vi "Read Command Error.vi"(8 "error in (no error)":errorcluster, 11 "VISA resource name":refnum<visa-resource-name>) -> (0 "error out":errorcluster, 1 "Error Message":string, 2 "Error Code":i32, 3 "VISA resource name out":refnum<visa-resource-name>)   [LabVIEW 2013, in "LeCroy Wave Series.lvlib"]
doc: "Reads and clears the contents of the Command error Register which specifies the last syntax error type detected by your oscilloscope."
uses:
  LeCroy Wave Series.lvlib
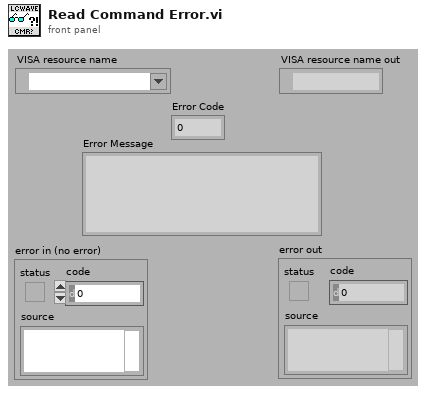
[diagram p1: front panel]
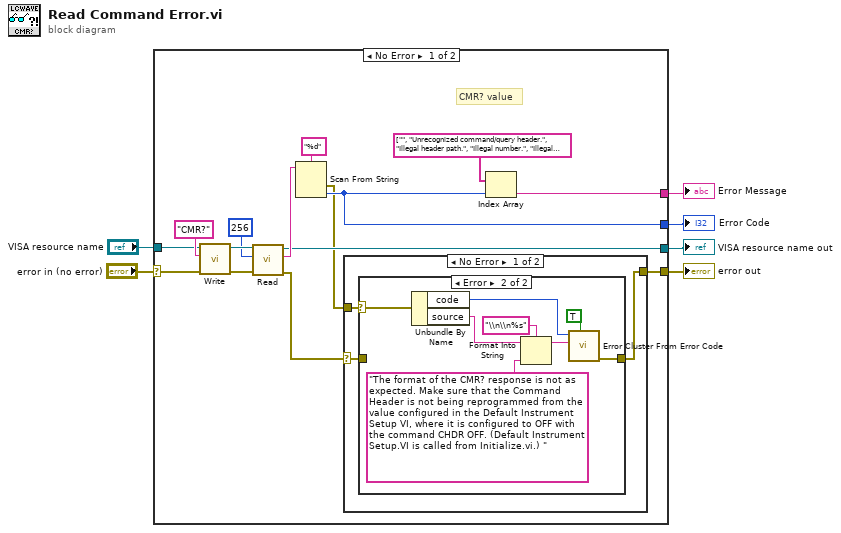
[diagram p0: block diagram]
diagram:
  n1 = case shown="No Error" "error in (no error)" {
    selector: "error in (no error)" -> [w8 w35]
    tunnel: [w14 _] -> w6
    tunnel: "VISA resource name" -> [w13 w36]
    tunnel: [w12 _] -> w4
    tunnel: [w11 w36] -> w3
    tunnel: [w9 w35] -> w2
    frame No Error {
      # "CMR? value"
      n2 = call "Write.vi"("error in (no error)"=w8, "Write Buffer"="CMR?" ("write buffer"), "VISA resource name"=w13) -> ("error out"=w20:errorcluster, "VISA resource name out"=w21:refnum<visa-resource-name>)  [unwired: 6 in, 1 out]
      n3 = call "Read.vi"("error in (no error)"=w20, "Byte Count"=u32 256 ("byte count"), "VISA resource name"=w21) -> ("error out"=w10:errorcluster, "Read Buffer"=w17:string, "VISA resource name out"=w11:refnum<visa-resource-name>)  [unwired: 5 in, 1 out]
      n4 = Scan From String(format string="%d", input string=w17) -> (error out=w7:errorcluster, output 1=w14:i32)  [unwired: 3 in, 2 out]
      n5 = case shown="No Error" w10 {
        selector: w10 -> [w24 w34]
        tunnel: [w23 w34] -> w9
        tunnel: w7 -> [w22 _]
        frame No Error {
          n6 = case shown="Error" w22 {
            selector: w22 -> [_ w29]
            tunnel: w24 -> [w25 _]
            tunnel: [w25 w32] -> w23
            frame No Error {
            }
            frame Error {
              n7 = Unbundle By Name(w29) -> ("code"=w28:i32, "source"=w27:string)
              n8 = Format Into String(format string="\\n\\n%s", initial string=w27, "The format of the CMR? response is not as expected. Make sure that the Command Header is not being reprogrammed from the value configured in the Default Instrument Setup VI, where it is configured to OFF with the command CHDR OFF. (Default Instrument Setup.VI is called from Initialize.vi.) " ("source")) -> (resulting string=w26:string)  [unwired: 1 in, 1 out]
              n9 = call <vilib>:"Error Cluster From Error Code.vi"("show call chain? (False)"=TRUE, "error message (\"\")"=w26, "error code (0)"=w28) -> ("error out"=w32:errorcluster)  [unwired: 6 in]
            }
          }
        }
        frame Error {
        }
      }
      n10 = Index Array(array=string[] ["", "Unrecognized command/query header.", "Illegal header path.", "Illegal number.", "Illegal number suffix.", "Unrecognized keyword.", "String error.", "GET embedded in another message.", "", "", "Arbitrary data block expected.", "Non-digit character in byte count field of arbitrary data block.", "EOI detected during definite length data block transfer.", "Extra bytes detected during definite length data block transfer."], index=w14) -> (element=w12:string)
    }
    frame Error {
    }
  }
  "Error Message" <- w4
  "Error Code" <- w6
  "VISA resource name out" <- w3
  "error out" <- w2
